vi "AutonVisionTrack2.vi"(3 "Refnum in":refnum<k33>) -> (10 "rt fifo out":refnum<k33>)   [LabVIEW 2014]
uses:
  TeleopCmd.ctl
  CmdFlag.ctl
  VisionInfoCluster.ctl
  Vision Data.vi
  encoderData.vi
  AutonCals.vi
panel:
  out "Waveform Chart 2":dbl(graph)
  out "Waveform Chart":dbl(graph)
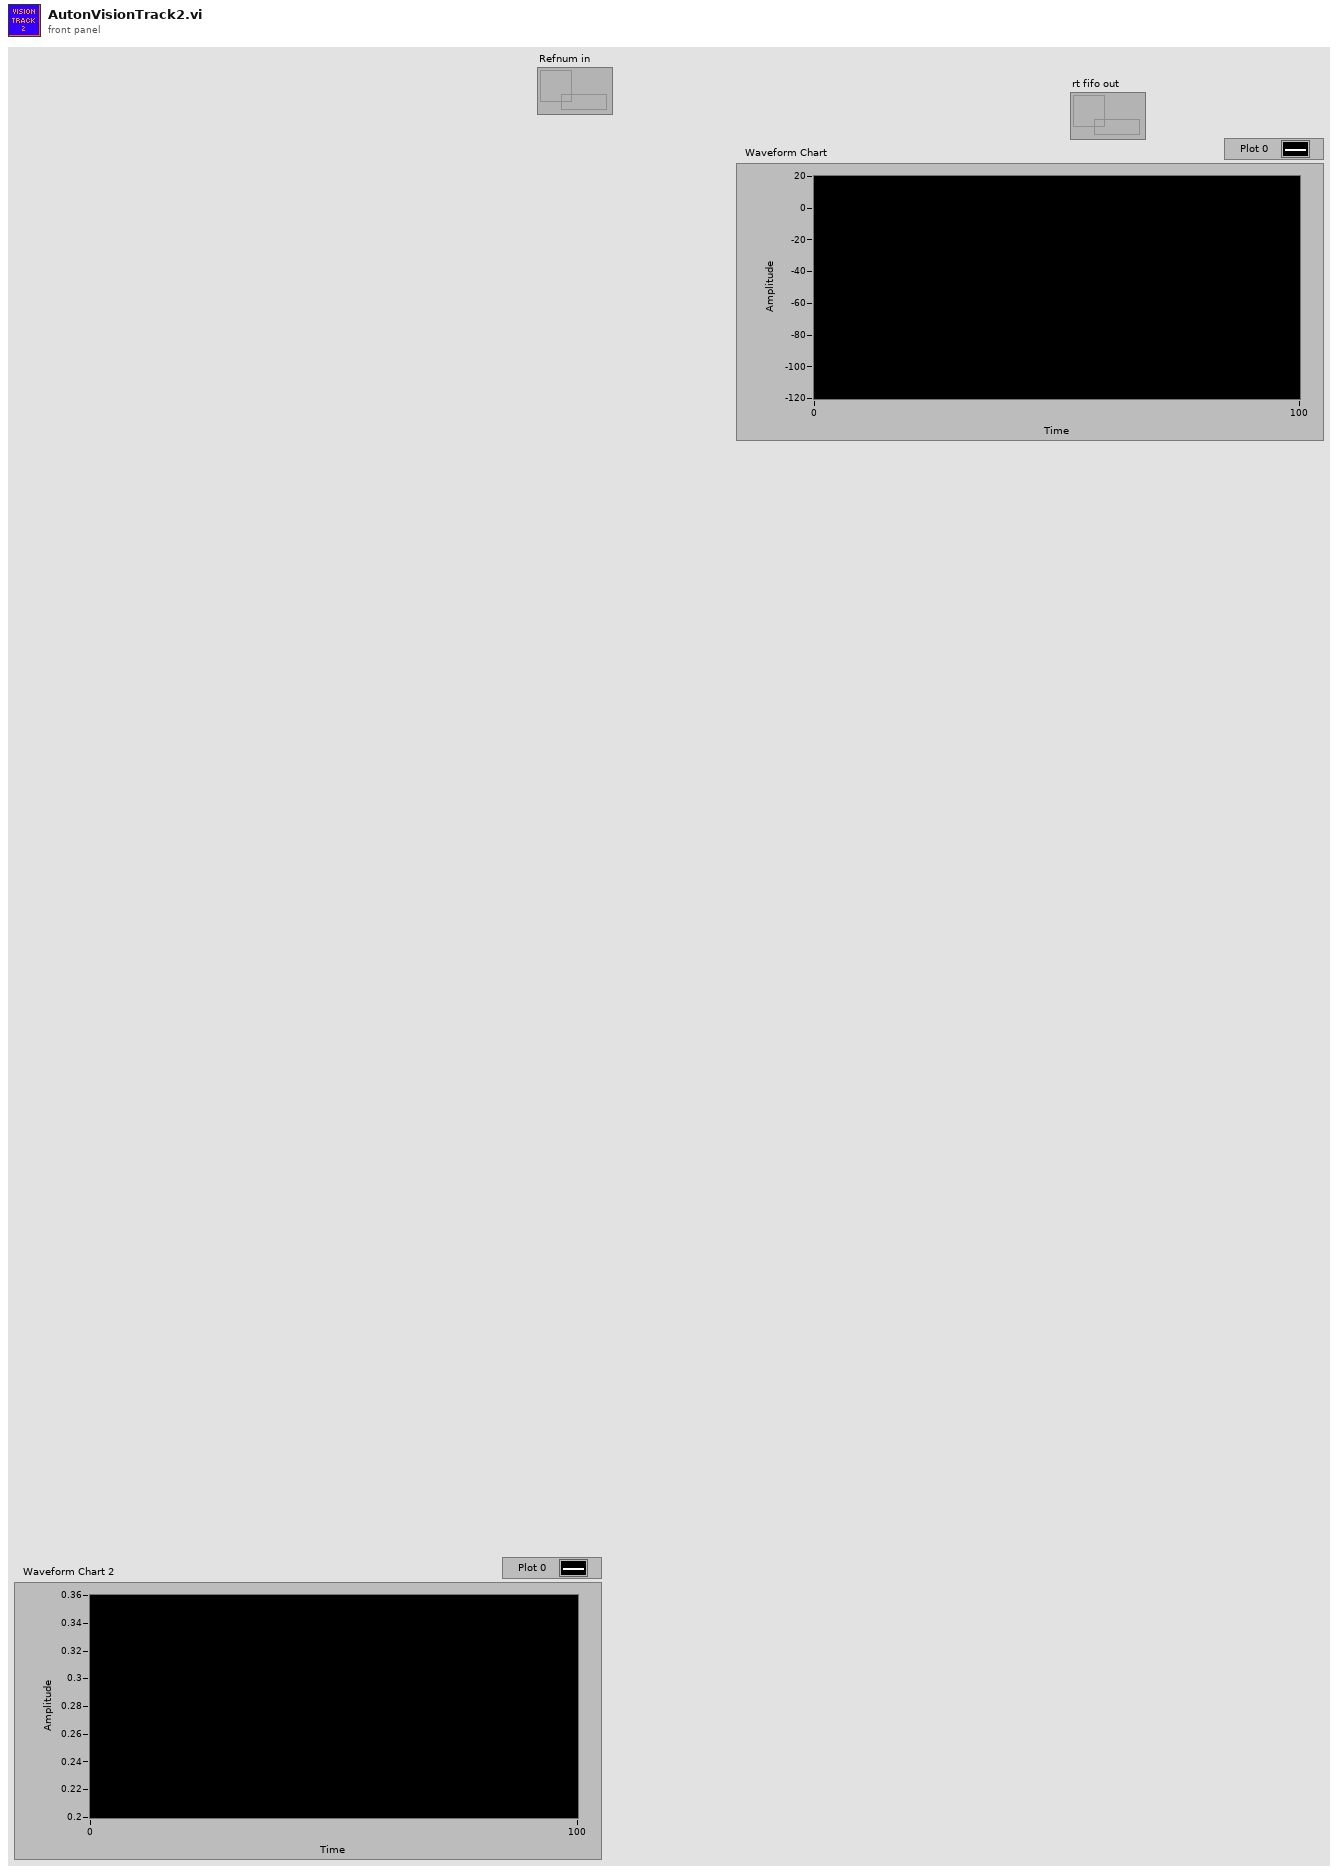
[diagram p1: front panel]
types:
  T1 = typedef "VisionInfoCluster.ctl" = cluster{"X":dbl, "Y":dbl}
  T2 = cluster{"proportional gain (Kc)":dbl, "integral time (Ti, min)":dbl, "derivative time (Td, min)":dbl}
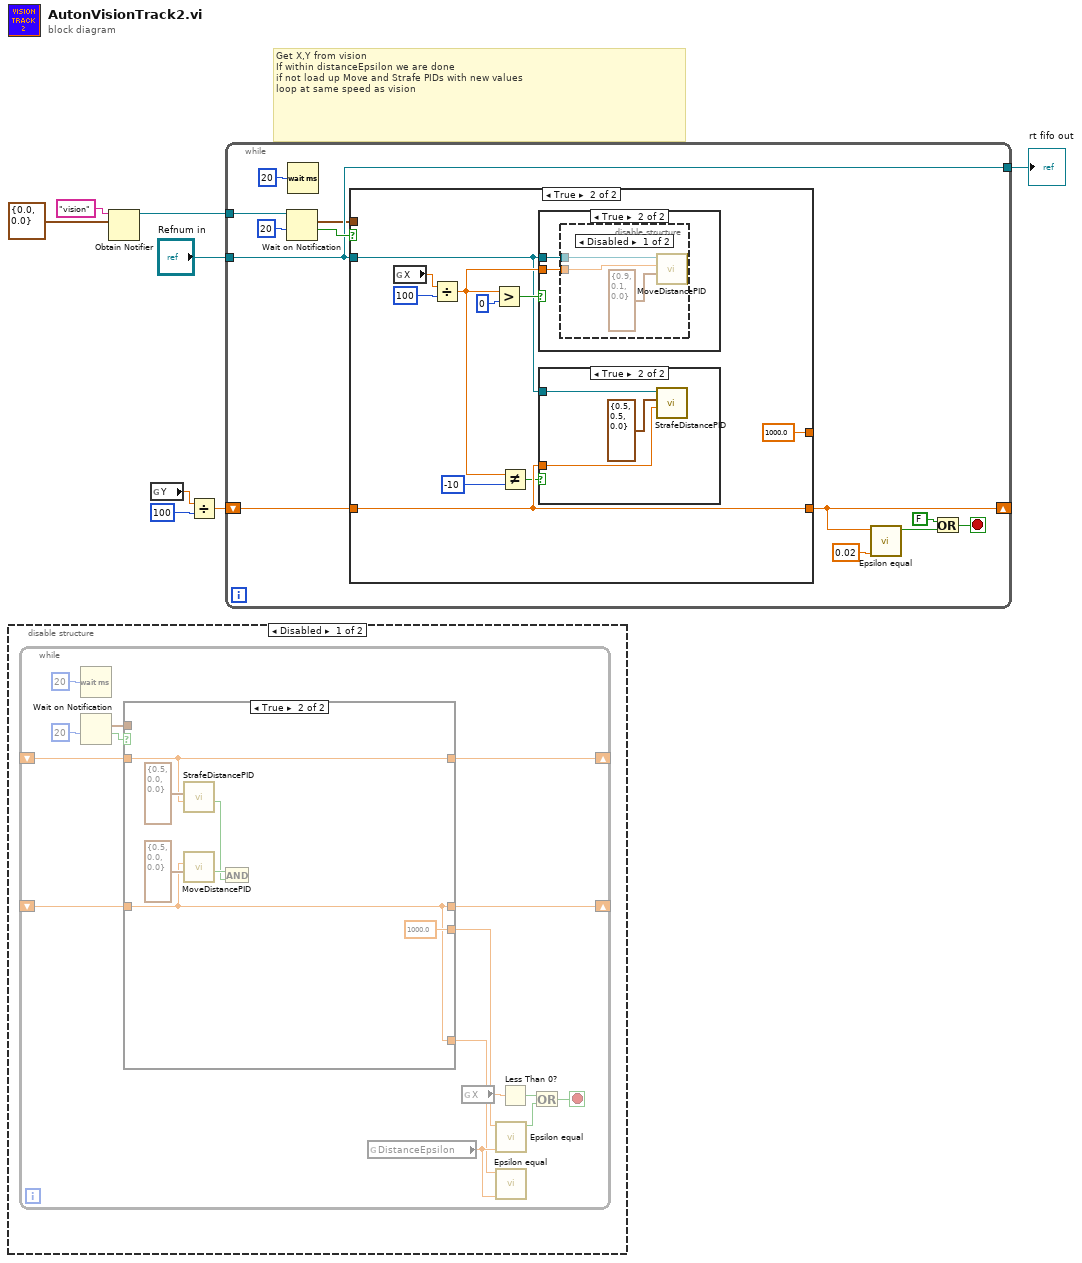
[diagram p0: block diagram]
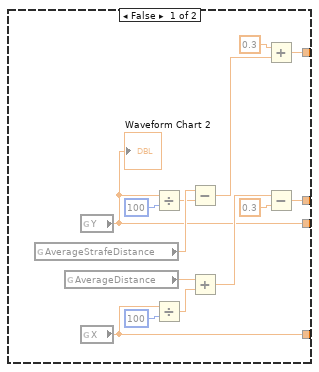
[diagram p2: hidden frame]
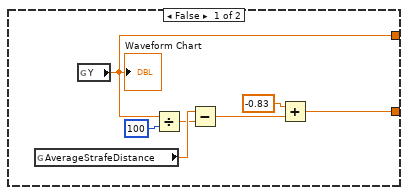
[diagram p4: hidden frame]
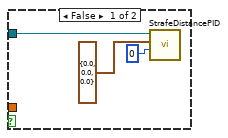
[diagram p5: hidden frame]
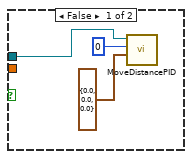
[diagram p6: hidden frame]
diagram:
  # "Get X,Y from vision\nIf within distanceEpsilon we are done\nif not load up Move and Strafe PIDs with new values\nloop at same speed as vision"
  n1 = disable-structure shown="Disabled" {
    frame Disabled {
      n2 = while {
        shift-right: [w20] -> _
        shift-left: _ -> [w19]
        shift-right: [w16] -> _
        shift-left: _ -> [w15]
        stop <- w9 stop-if-true
        n3 = Wait (ms)(milliseconds to wait=u32 20) -> ()  [unwired: 1 out]
        n4 = Wait on Notification(timeout in ms (-1)=20) -> (notification=w21:T1, timed out?=w22:bool)  [unwired: 3 in, 2 out]
        n5 = case shown="True" w22 {
          tunnel: w21 -> [_ _]
          tunnel: [w26 w38] -> w20
          tunnel: w19 -> [_ w38]
          tunnel: [w24 1000.0 ("Y")] -> w18
          tunnel: [w29 w39] -> w16
          tunnel: w15 -> [_ w39]
          tunnel: [w25 w39] -> w13
          frame False {
            n6 = global read "encoderData.vi" "AverageStrafeDistance"() -> (w36:dbl)
            n7 = global read "encoderData.vi" "AverageDistance"() -> (w33:dbl)
            n8 = global read "Vision Data.vi" "Y"() -> (w24:dbl)
            "Waveform Chart 2" <- w24
            n9 = global read "Vision Data.vi" "X"() -> (w25:dbl)
            n10 = Divide(x=w24, y=100) -> (x/y=w35:dbl)
            n11 = Divide(x=w25, y=100) -> (x/y=w32:dbl)
            n12 = Subtract(x=w36, y=w35) -> (x-y=w28:dbl)
            n13 = Add(x=w33, y=w32) -> (x+y=w31:dbl)
            n14 = Add(x=0.3, y=w28) -> (x+y=w26:dbl)
            n15 = Subtract(x=w31, y=0.3) -> (x-y=w29:dbl)
          }
          frame True {
            n16 = call "StrafeDistancePID.vi"("Distance"=w38, "PID gains"=T2 {"proportional gain (Kc)"=0.5, "integral time (Ti, min)"=0.0, "derivative time (Td, min)"=0.0}) -> ("Boolean"=w42:bool)  [unwired: 7 in, 2 out]
            n17 = call "MoveDistancePID.vi"("PID gains"=T2 {"proportional gain (Kc)"=0.5, "integral time (Ti, min)"=0.0, "derivative time (Td, min)"=0.0}, "Distance"=w39) -> ("Boolean"=w43:bool)  [unwired: 7 in, 2 out]
            n18 = And(x=w43, y=w42) -> ()  [unwired: 1 out]
          }
        }
        n19 = global read "AutonCals.vi" "DistanceEpsilon"() -> (w14:dbl)
        n20 = global read "Vision Data.vi" "X"() -> (w12:dbl)
        n21 = call "Epsilon equal.vi"("Epsilon"=w14, "Value1"=w18) -> ("Boolean"=w10:bool)  [unwired: 9 in]
        n22 = call "Epsilon equal.vi"("Epsilon"=w14, "Value1"=w13) -> ()  [unwired: 9 in, 1 out]
        n23 = Less Than 0?(x=w12) -> (x < 0?=w11:bool)
        n24 = Or(x=w11, y=w10) -> (x .or. y?=w9:bool)
      }
    }
    frame Enabled {
    }
  }
  n25 = Obtain Notifier(name (unnamed)="vision", notification data type=T1 {"X"=0.0, "Y"=0.0}) -> (notifier out=w6:refnum<notifier>)  [unwired: 2 in, 2 out]
  n26 = global read "Vision Data.vi" "Y"() -> (w2:dbl)
  n27 = Divide(x=w2, y=100) -> (x/y=w1:dbl)
  n28 = while {
    tunnel: w6 -> [w56]
    tunnel: "Refnum in" -> [w53]
    tunnel: [w53] -> w4
    shift-right: [w46] -> _
    shift-left: w1 -> [w50]
    stop <- w48 stop-if-true
    n29 = Wait on Notification(notifier=w56, timeout in ms (-1)=20) -> (notification=w52:T1, timed out?=w54:bool)  [unwired: 2 in, 2 out]
    n30 = Wait (ms)(milliseconds to wait=u32 20) -> ()  [unwired: 1 out]
    n31 = case shown="True" w54 {
      tunnel: w53 -> [_ w64]
      tunnel: w52 -> [_ _]
      tunnel: [w58 1000.0 ("Y")] -> _
      tunnel: [w57 w72] -> w46
      tunnel: w50 -> [_ w72]
      frame False {
        n32 = global read "encoderData.vi" "AverageStrafeDistance"() -> (w62:dbl)
        n33 = global read "Vision Data.vi" "Y"() -> (w58:dbl)
        "Waveform Chart" <- w58
        n34 = Divide(x=w58, y=100) -> (x/y=w61:dbl)
        n35 = Subtract(x=w62, y=w61) -> (x-y=w60:dbl)
        n36 = Add(x=-0.83, y=w60) -> (x+y=w57:dbl)
      }
      frame True {
        n37 = global read "Vision Data.vi" "X"() -> (w69:dbl)
        n38 = Divide(x=w69, y=100) -> (x/y=w67:dbl)
        n39 = Greater?(x=w67, y=0) -> (0:w70:bool)
        n40 = Not Equal?(x=w67, y=-10) -> (x != y?=w65:bool)
        n41 = case shown="True" w70 {
          tunnel: w64 -> [w82 w84]
          tunnel: w67 -> [_ w83]
          frame False {
            n42 = call "MoveDistancePID.vi"("PID gains"=T2 {"proportional gain (Kc)"=0.0, "integral time (Ti, min)"=0.0, "derivative time (Td, min)"=0.0}, "Distance"=0, "Refnum in"=w82) -> ()  [unwired: 6 in, 3 out]
          }
          frame True {
            n43 = disable-structure shown="Disabled" {
              disable-tunnel: w84 -> [w87 _]
              disable-tunnel: w83 -> [w86 _]
              frame Disabled {
                n44 = call "MoveDistancePID.vi"("PID gains"=T2 {"proportional gain (Kc)"=0.9, "integral time (Ti, min)"=0.1, "derivative time (Td, min)"=0.0}, "Distance"=w86, "Refnum in"=w87) -> ()  [unwired: 6 in, 3 out]
              }
              frame Enabled {
              }
            }
          }
        }
        n45 = case shown="True" w65 {
          tunnel: w72 -> [_ w78]
          tunnel: w64 -> [w74 w77]
          frame False {
            n46 = call "StrafeDistancePID.vi"("Distance"=0, "PID gains"=T2 {"proportional gain (Kc)"=0.0, "integral time (Ti, min)"=0.0, "derivative time (Td, min)"=0.0}, "Refnum in"=w74) -> ()  [unwired: 6 in, 3 out]
          }
          frame True {
            n47 = call "StrafeDistancePID.vi"("Distance"=w78, "PID gains"=T2 {"proportional gain (Kc)"=0.5, "integral time (Ti, min)"=0.5, "derivative time (Td, min)"=0.0}, "Refnum in"=w77) -> ()  [unwired: 6 in, 3 out]
          }
        }
      }
    }
    n48 = call "Epsilon equal.vi"("Epsilon"=0.02 ("Value2"), "Value1"=w46) -> ("Boolean"=w49:bool)  [unwired: 9 in]
    n49 = Or(x=FALSE, y=w49) -> (x .or. y?=w48:bool)
  }
  "rt fifo out" <- w4
